vi "Camera_control_v4.vi"() -> ()   [LabVIEW 2018]
uses:
  System.Windows.Forms
  C:/Program Files/National Instruments/LabVIEW 2018/uc480DotNet.dll
  uc480DotNet.dll
panel:
  out "Time Stamp 5":timestamp format="%<%H:%M:%S\n%Y/%m/%d>T"
  out "Time Stamp 2":timestamp format="%<%H:%M:%S\n%Y/%m/%d>T"
  out "Boolean":bool
  out "?":u8(slide) scale=0.0..1.0
  in  "Capture Period (hours) 2":dbl=0.005
  in  "stop":bool
  out "Image":picture
  in  "Capture Frequency (minutes)":dbl=0.5
  out "Time Stamp":timestamp format="%<%H:%M:%S\n%Y/%m/%d>T"
  in  "Name of Operator":string="AT"
  in  "Parent Folder":path=path "D:/Dropbox (MIT)/Buonassisi-Group/AMD Team/Campaign 2.0/Degradation"
  in  "Zoom":u16(ring)=1 items=["4X"=4, "2X"=2, "1X"=1]
  in  "PictureBox":refnum<k24>(container)
  out "Serial Number 2":string
  out "Height 2":i32=8
  out "Width 2":i32=8
  out "Bits/Pixel 2":i32=8
  in  "Camera ID":i32
  out "Serial Number":string
  out "Height":i32=8
  out "Width":i32=8
  out "Bits/Pixel":i32=8
  in  "Pixelclock":i32(slide)=33 min=5 max=40 step=1 scale=5.0..40.0
  in  "Framerate":dbl(slide)=33.21525 min=0.47411700449083627 max=15.001275108384213 step=0.014032998230479876 scale=0.47411700449083627..15.001275108384213 scale format="%#.3g"
  in  "Exposure":dbl(slide)=33.21525 min=0.06241666666666667 max=99.86666666666667 step=0.06241666666666667 scale=0.06241666666666667..99.86666666666667 scale format="%#.3g"
  out "Error Out":errorcluster caption="error"
  in  "Load Parameter":bool
  in  "Exit Camera":bool
  in  "Stop Live":bool
  in  "Start Live":bool
  in  "Init Camera":bool
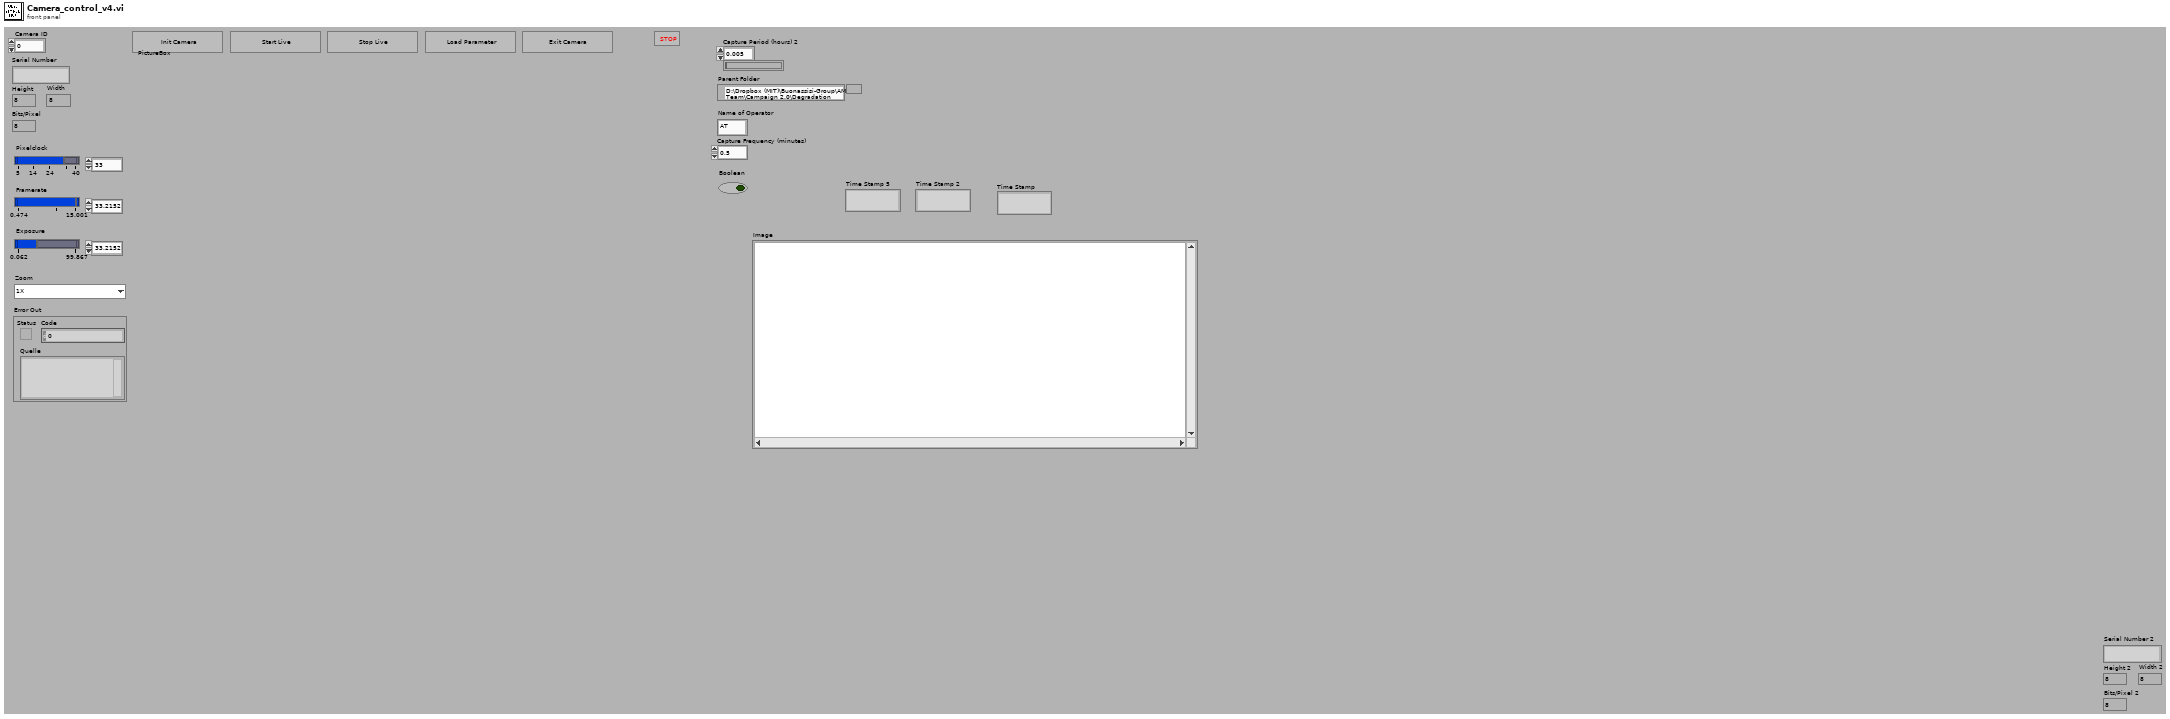
[diagram p1: front panel]
types:
  T1 = enum8{"Enabled", "Disabled", "Disabled and Grayed Out"}
  T2 = typedef "imagedata.ctl" = cluster{"image type":i32, "image depth":i32, "image":u8[], "mask":u8[], "colors":u32[], "Rectangle":cluster{"left":i16, "top":i16, "right":i16, "bottom":i16}}
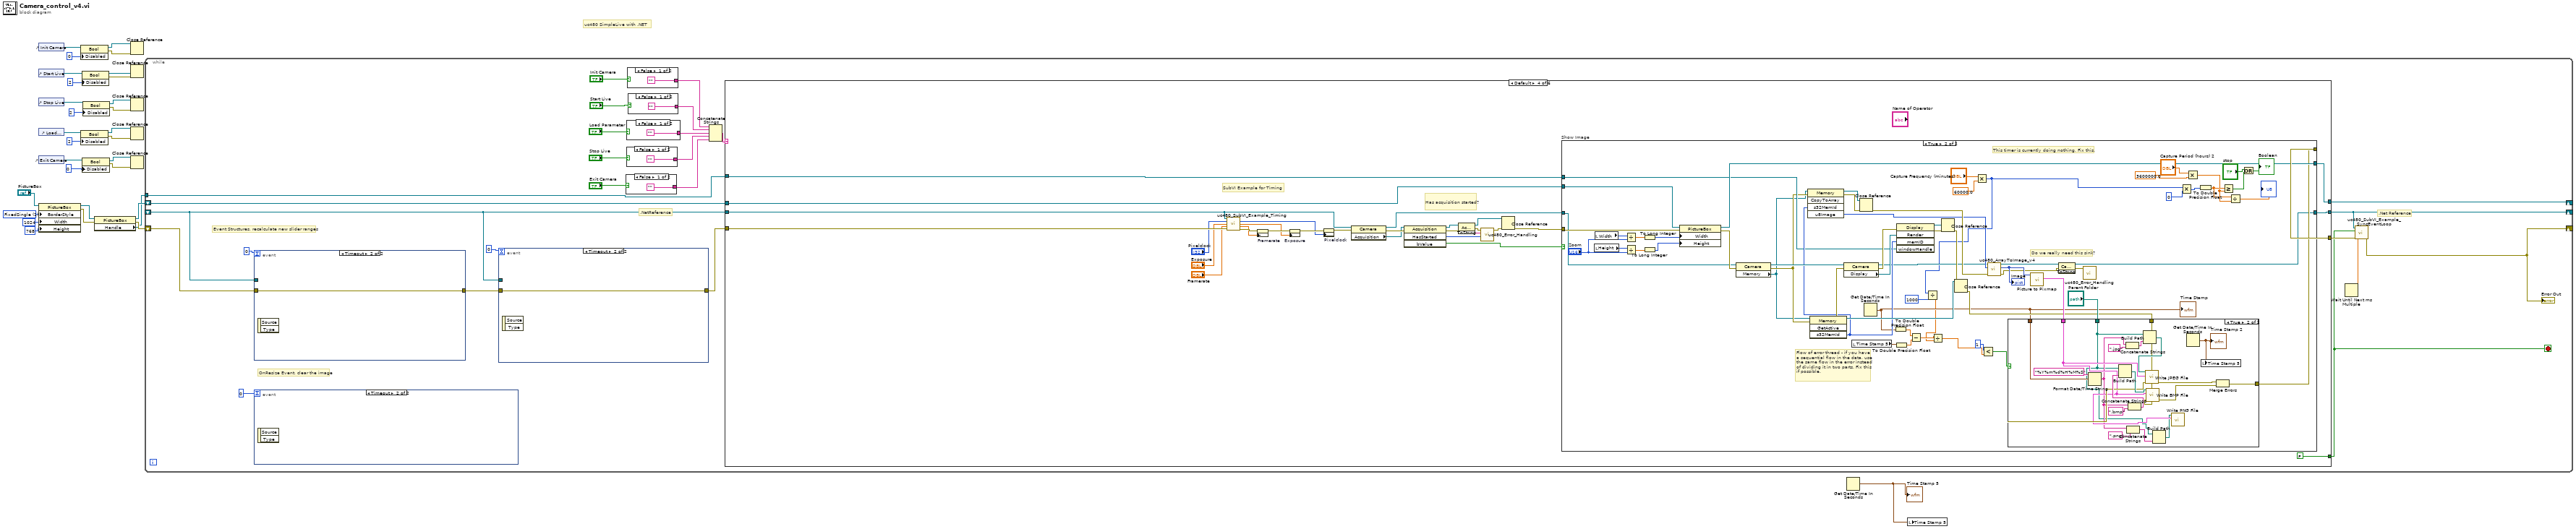
[diagram p0: block diagram]
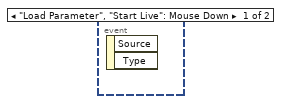
[diagram p2: hidden frame]
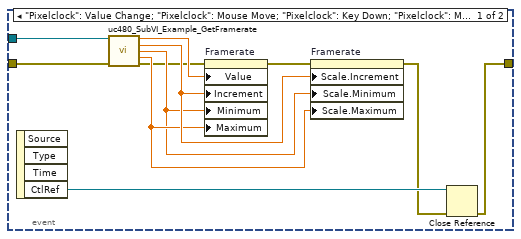
[diagram p3: hidden frame]
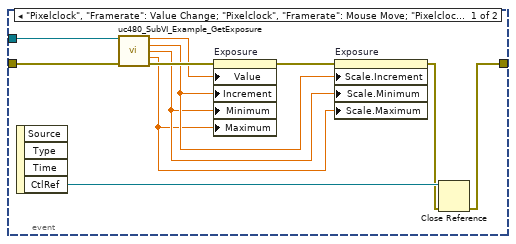
[diagram p4: hidden frame]
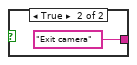
[diagram p5: hidden frame]
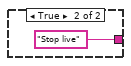
[diagram p6: hidden frame]
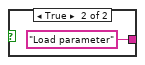
[diagram p7: hidden frame]
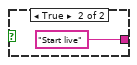
[diagram p8: hidden frame]
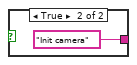
[diagram p9: hidden frame]
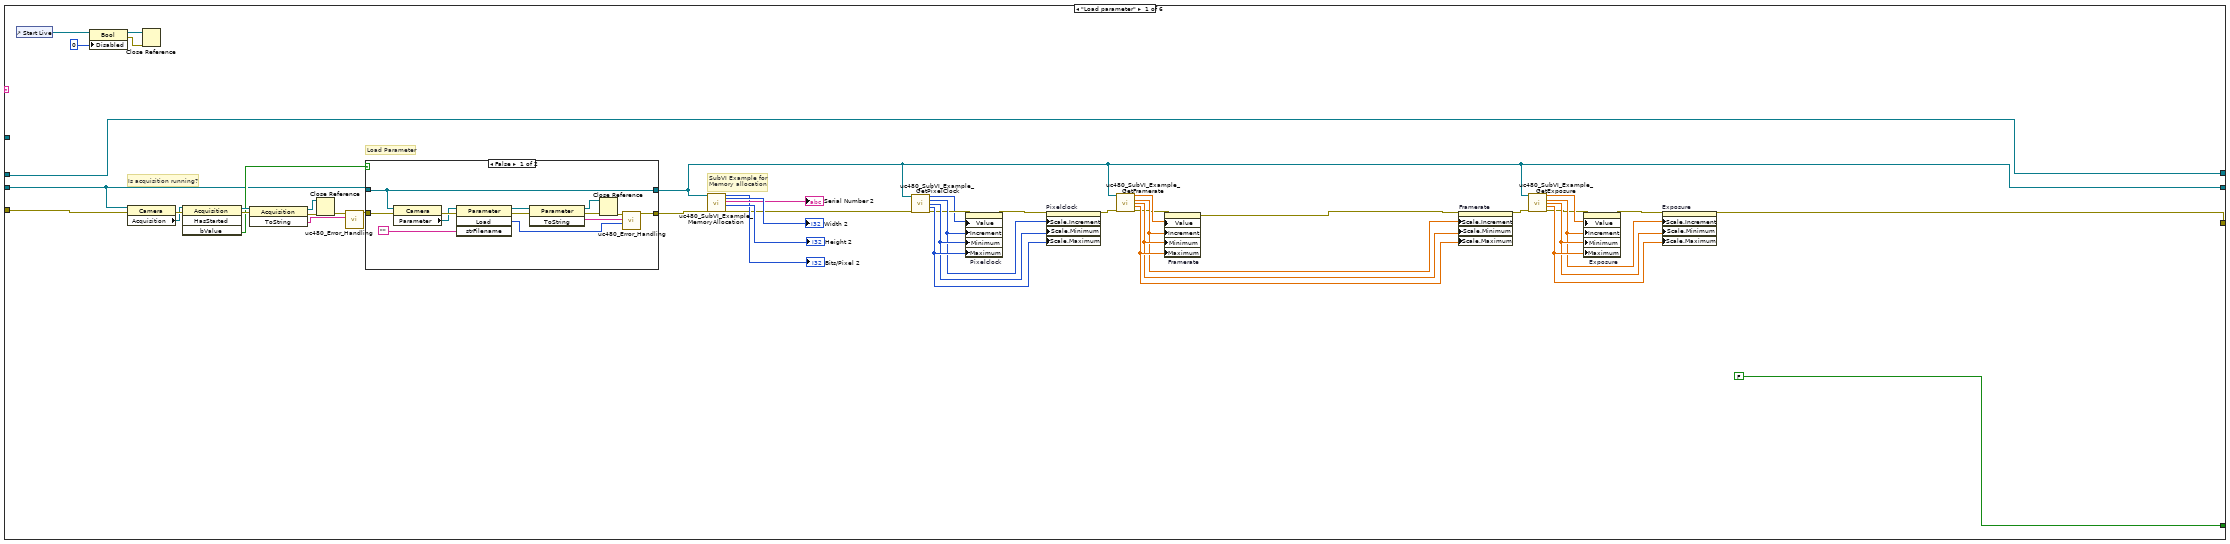
[diagram p10: hidden frame]
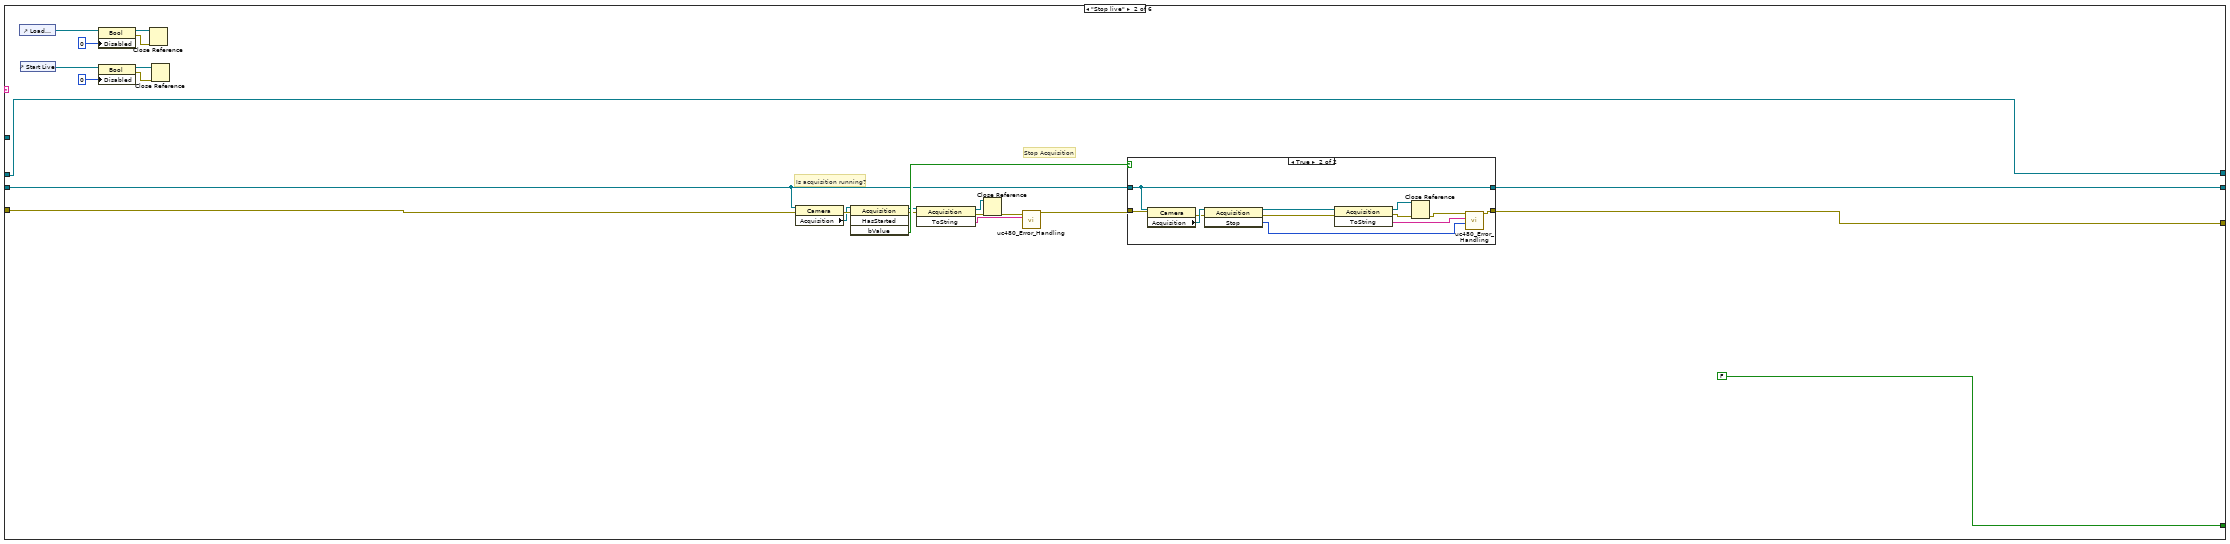
[diagram p12: hidden frame]
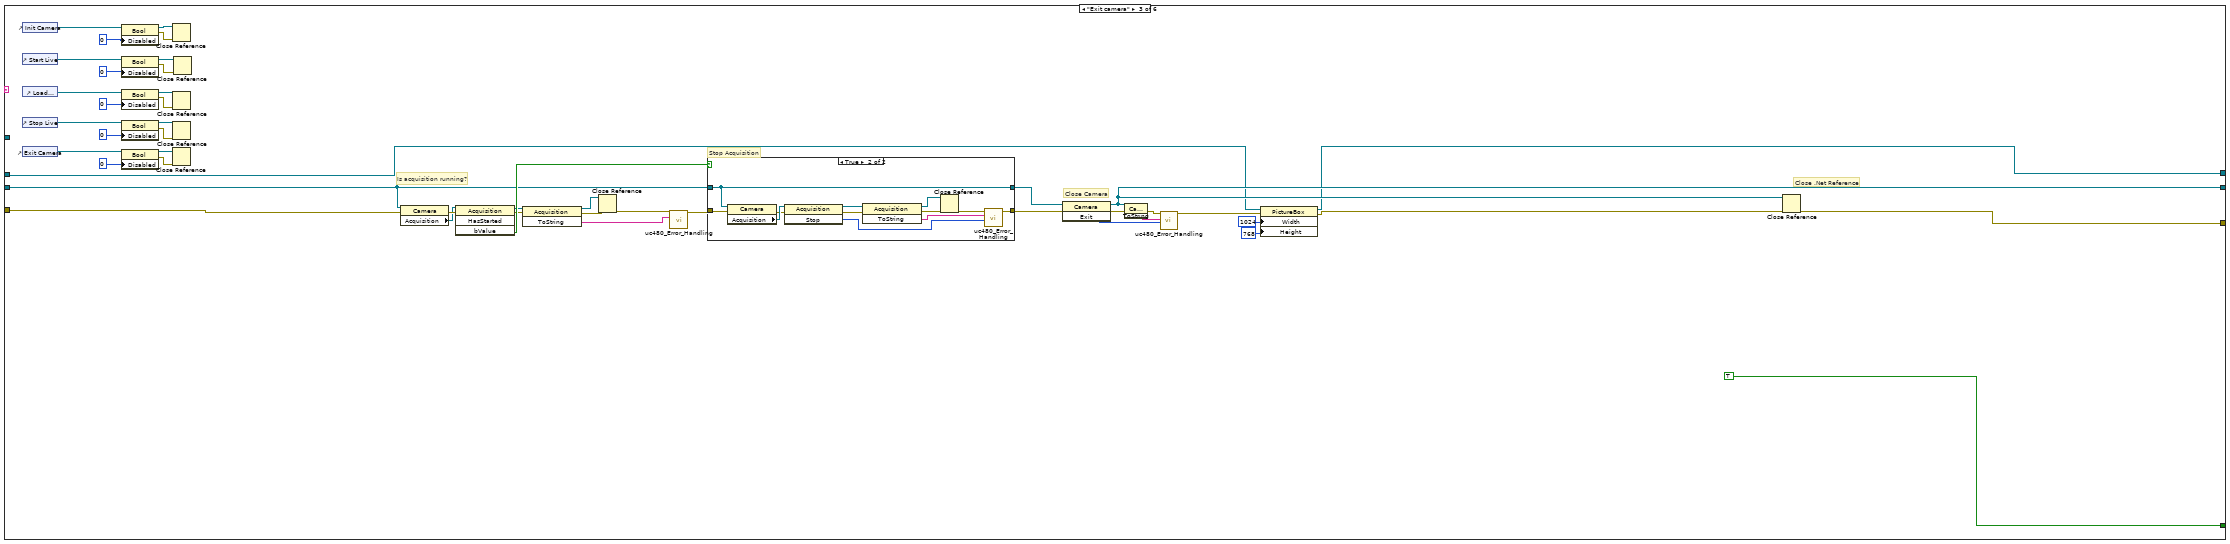
[diagram p14: hidden frame]
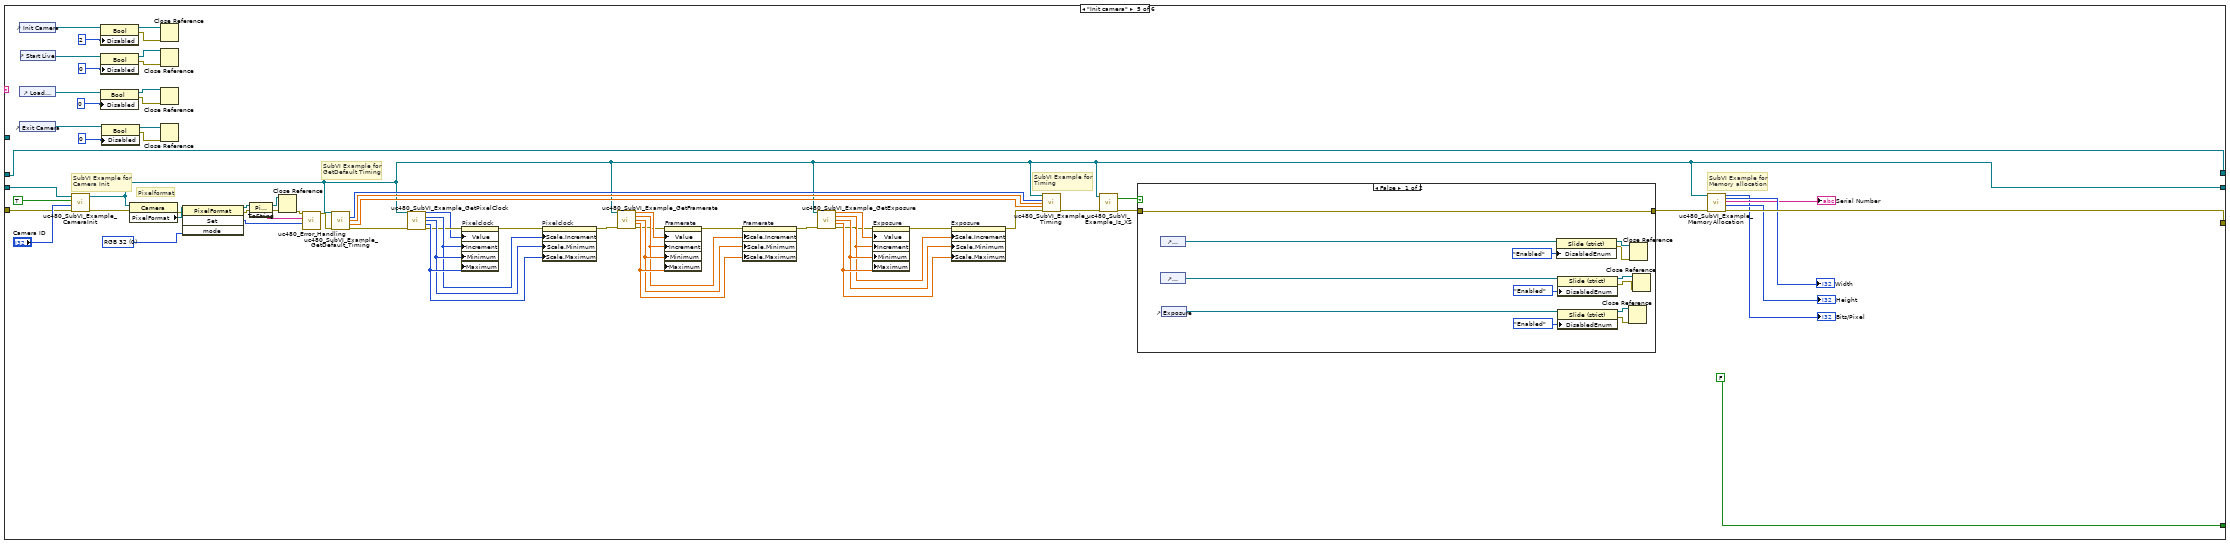
[diagram p18: hidden frame]
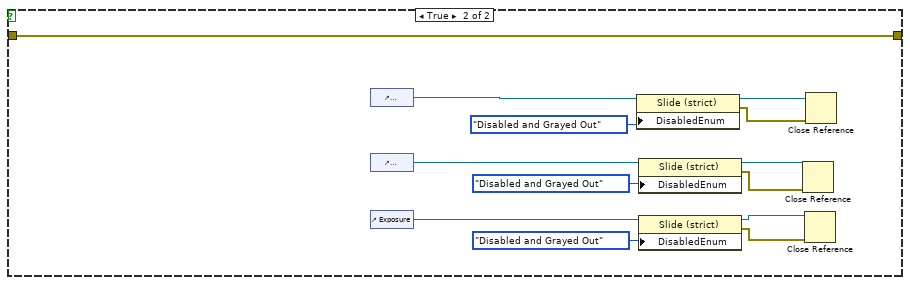
[diagram p19: hidden frame]
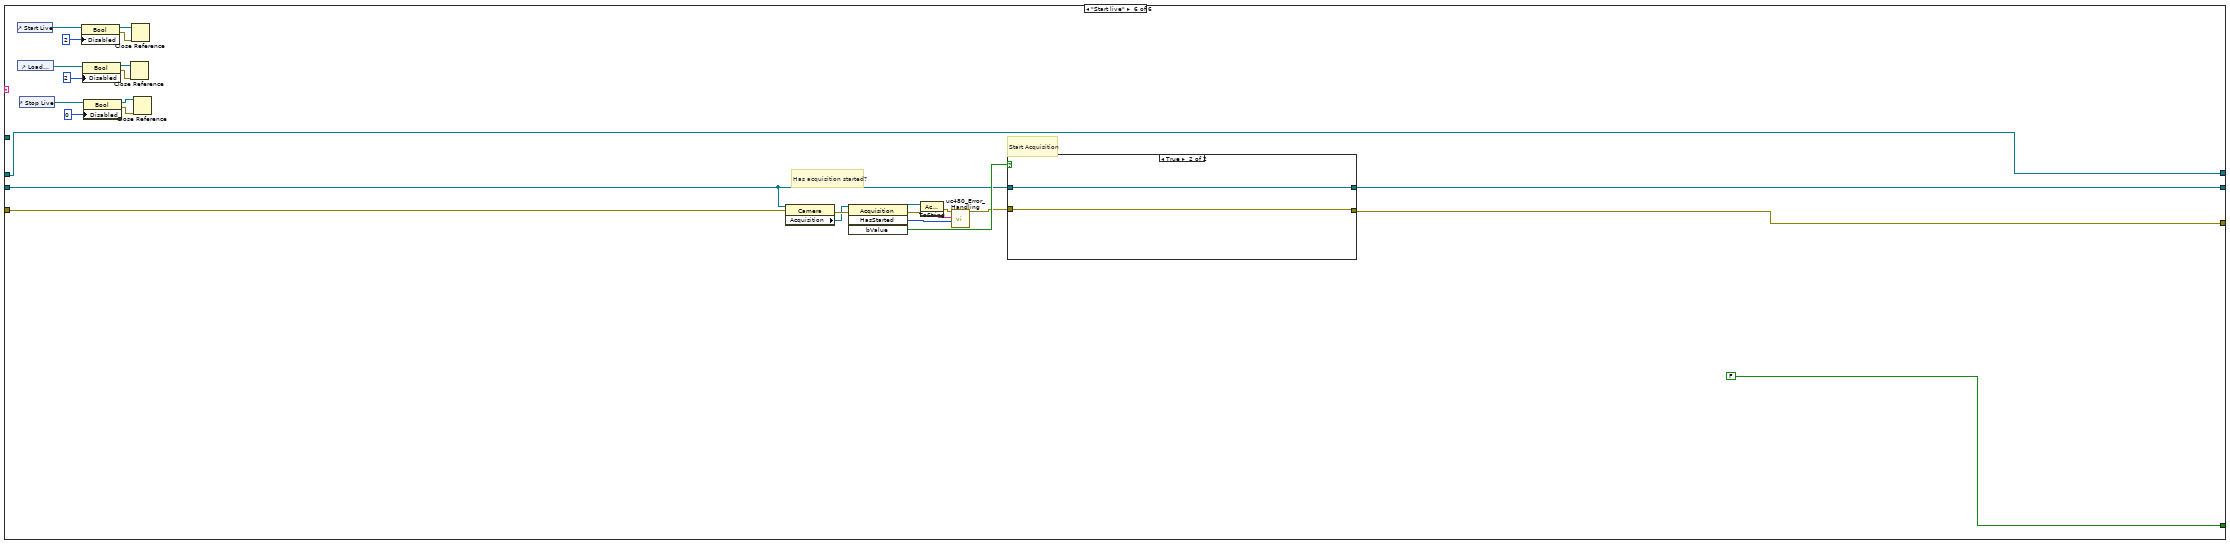
[diagram p20: hidden frame]
diagram:
  w19 = 1 items=["None", "FixedSingle", "Fixed3D"] ("BorderStyle")
  # "uc480 SimpleLive with .NET"
  n1 = control-ref of="Init Camera"() -> (w30:refnum<vi>)
  n2 = control-ref of="Start Live"() -> (w27:refnum<vi>)
  n3 = control-ref of="Stop Live"() -> (w21:refnum<vi>)
  n4 = control-ref of="Load Parameter"() -> (w22:refnum<vi>)
  n5 = control-ref of="Exit Camera"() -> (w23:refnum<vi>)
  n6 = property class="PictureBox"(reference="PictureBox", "BorderStyle"=w19, "Width"=1024, "Height"=768) -> (reference out=w5:refnum<k24>, error out=w6:errorcluster)  [unwired: 1 in]
  n7 = property class="Bool"(reference=w30, "Disabled"=u8 0 ("Deaktiviert")) -> (reference out=w16:refnum<vi>, error out=w15:errorcluster)  [unwired: 1 in]
  n8 = property class="Bool"(reference=w22, "Disabled"=u8 2 ("Deaktiviert")) -> (reference out=w10:refnum<vi>, error out=w9:errorcluster)  [unwired: 1 in]
  n9 = property class="Bool"(reference=w27, "Disabled"=u8 2 ("Deaktiviert")) -> (reference out=w14:refnum<vi>, error out=w13:errorcluster)  [unwired: 1 in]
  n10 = property class="Bool"(reference=w23, "Disabled"=u8 0 ("Deaktiviert")) -> (reference out=w8:refnum<vi>, error out=w7:errorcluster)  [unwired: 1 in]
  n11 = property class="Bool"(reference=w21, "Disabled"=u8 2 ("Deaktiviert")) -> (reference out=w12:refnum<vi>, error out=w11:errorcluster)  [unwired: 1 in]
  n12 = property class="PictureBox"(reference=w5, error in=w6) -> (reference out=w4:refnum<k24>, error out=w3:errorcluster, "Handle"=w2:refnum<k24>)
  n13 = Close Reference(reference=w16, error in (no error)=w15) -> ()  [unwired: 1 out]
  n14 = Close Reference(reference=w14, error in (no error)=w13) -> ()  [unwired: 1 out]
  n15 = Close Reference(reference=w12, error in (no error)=w11) -> ()  [unwired: 1 out]
  n16 = Close Reference(reference=w10, error in (no error)=w9) -> ()  [unwired: 1 out]
  n17 = Close Reference(reference=w8, error in (no error)=w7) -> ()  [unwired: 1 out]
  n18 = while {
    shift-right: [w36] -> _
    shift-left: w3 -> [w41]
    shift-right: [w39] -> _
    shift-left: _ -> [w32]
    shift-right: [w34] -> _
    shift-left: w4 -> [w35]
    tunnel: w2 -> [w33]
    stop <- w31 stop-if-true
    # "OnResize Event, clear the image"
    # "Event Structures, recalculate new slider ranges"
    # ".NetReference"
    # ".Net Reference"
    n19 = event shown="[1] Timeout" {
      selector: _ -> [_ _]
      dyn-events: _ -> [_ _]
      timeout: 0 -> [_ _]
      tunnel: [w57 w68] -> w42
      tunnel: w41 -> [w67 w68]
      tunnel: w32 -> [w66 _]
      event "Pixelclock": Value Change; "Pixelclock": Mouse Move; "Pixelclock": Key Down; "Pixelclock": Mouse Up {
        n20 = event-data() -> ("CtlRef"=w59:refnum<vi>)  [unwired: 1 in, 3 out]
        n21 = call <instrlib>:"uc480_SubVI_Example_GetFramerate.vi"(".NET (Reference)"=w66, "Error In"=w67) -> ("Framerate"=w65:dbl, "Inc"=w64:dbl, "Min"=w62:dbl, "Max"=w63:dbl, "error out"=w61:errorcluster)  [unwired: 9 in]
        n22 = property on="Framerate" class="Slide (strict)"(error in=w61, "Value"=w65, "Increment"=w64, "Minimum"=w62, "Maximum"=w63) -> (error out=w60:errorcluster)  [unwired: 1 in, 1 out]
        n23 = property on="Framerate" class="Slide (strict)"(error in=w60, "Scale.Increment"=w64, "Scale.Minimum"=w62, "Scale.Maximum"=w63) -> (error out=w58:errorcluster)  [unwired: 1 in, 1 out]
        n24 = Close Reference(reference=w59, error in (no error)=w58) -> (error out=w57:errorcluster)
      }
      event Timeout {
        n25 = event-data() -> ()  [unwired: 1 in, 2 out]
      }
    }
    n26 = event shown="[1] Timeout" {
      selector: _ -> [_ _]
      dyn-events: _ -> [_ _]
      timeout: 0 -> [_ _]
      event "Load Parameter", "Start Live": Mouse Down {
        n27 = event-data() -> ()  [unwired: 1 in, 2 out]
      }
      event Timeout {
        n28 = event-data() -> ()  [unwired: 1 in, 2 out]
      }
    }
    n29 = event shown="[1] Timeout" {
      selector: _ -> [_ _]
      dyn-events: _ -> [_ _]
      timeout: 0 -> [_ _]
      tunnel: w42 -> [w79 w80]
      tunnel: [w69 w80] -> w44
      tunnel: w32 -> [w78 _]
      event "Pixelclock", "Framerate": Value Change; "Pixelclock", "Framerate": Mouse Move; "Pixelclock", "Framerate": Key Down; "Pixelclock", "Framerate": Mouse Up {
        n30 = event-data() -> ("CtlRef"=w71:refnum<vi>)  [unwired: 1 in, 3 out]
        n31 = call <instrlib>:"uc480_SubVI_Example_GetExposure.vi"(".NET (Reference)"=w78, "Error In"=w79) -> ("Exposure"=w75:dbl, "Inc"=w74:dbl, "Min"=w73:dbl, "Max"=w72:dbl, "Error out"=w76:errorcluster)  [unwired: 9 in]
        n32 = property on="Exposure" class="Slide (strict)"(error in=w76, "Value"=w75, "Increment"=w74, "Minimum"=w73, "Maximum"=w72) -> (error out=w77:errorcluster)  [unwired: 1 in, 1 out]
        n33 = property on="Exposure" class="Slide (strict)"(error in=w77, "Scale.Increment"=w74, "Scale.Minimum"=w73, "Scale.Maximum"=w72) -> (error out=w70:errorcluster)  [unwired: 1 in, 1 out]
        n34 = Close Reference(reference=w71, error in (no error)=w70) -> (error out=w69:errorcluster)
      }
      event Timeout {
        n35 = event-data() -> ()  [unwired: 1 in, 2 out]
      }
    }
    n36 = case shown="False" "Exit Camera" {
      tunnel: ["" "Exit camera"] -> w46
      frame False {
      }
      frame True {
      }
    }
    n37 = case shown="False" "Load Parameter" {
      tunnel: ["" "Load parameter"] -> w50
      frame False {
      }
      frame True {
      }
    }
    n38 = case shown="False" "Stop Live" {
      tunnel: ["" "Stop live"] -> w49
      frame False {
      }
      frame True {
      }
    }
    n39 = case shown="False" "Init Camera" {
      tunnel: ["" "Init camera"] -> w54
      frame False {
      }
      frame True {
      }
    }
    n40 = case shown="False" "Start Live" {
      tunnel: ["" "Start live"] -> w53
      frame False {
      }
      frame True {
      }
    }
    n41 = Concatenate Strings(w54, w53, w50, w49, w46) -> (w52:string)
    n42 = case shown="Default" w52 {
      tunnel: w32 -> [w127 w167 w221 w263 w425 w476]
      tunnel: w44 -> [w130 w168 w222 w273 w424 w477]
      tunnel: [w97 w166 w230 w272 w381 w475] -> w39
      tunnel: [w98 w165 w231 w271 w420 w473] -> w38
      tunnel: [FALSE FALSE TRUE FALSE FALSE FALSE] -> w31
      tunnel: w35 -> [w96 w159 w201 w255 w376 w466]
      tunnel: [w96 w159 w200 w254 w376 w466] -> w34
      tunnel: w33 -> [_ _ _ w251 _ _]
      frame "Load parameter" {
        # "SubVI Example for \nMemory allocation"
        # "Is acquisition running?"
        # "Load Parameter"
        n43 = control-ref of="Start Live"() -> (w121:refnum<vi>)
        n44 = property class="Bool"(reference=w121, "Disabled"=u8 0 ("Deaktiviert")) -> (reference out=w95:refnum<vi>, error out=w94:errorcluster)  [unwired: 1 in]
        n45 = property class="Camera"(reference=w127, error in=w130) -> (error out=w135:errorcluster, "Acquisition"=w134:refnum<k24>)  [unwired: 1 out]
        n46 = Close Reference(reference=w95, error in (no error)=w94) -> ()  [unwired: 1 out]
        n47 = invoke class="Acquisition" method="HasStarted"(reference=w134, error in=w135) -> (reference out=w131:refnum<k24>, error out=w133:errorcluster, "bValue"=w129:bool)  [unwired: 2 in, 1 out]
        n48 = invoke class="Acquisition" method="ToString"(reference=w131, error in=w133) -> (reference out=w93:refnum<k24>, error out=w92:errorcluster, "ToString"=w132:string)  [unwired: 1 in]
        n49 = Close Reference(reference=w93, error in (no error)=w92) -> (error out=w91:errorcluster)
        n50 = call <instrlib>:"uc480_Error_Handling.vi"("Error String"=w132, "Error In"=w91) -> ("Error Out"=w128:errorcluster)  [unwired: 9 in]
        n51 = case shown="False" w129 {
          tunnel: w128 -> [w143 w150]
          tunnel: w127 -> [w141 w151]
          tunnel: [w142 w150] -> w122
          tunnel: [w141 w151] -> w97
          frame False {
            n52 = property class="Camera"(reference=w141, error in=w143) -> (error out=w145:errorcluster, "Parameter"=w144:refnum<k24>)  [unwired: 1 out]
            n53 = invoke class="Parameter" method="Load"(reference=w144, error in=w145, "strFilename"="") -> (reference out=w147:refnum<k24>, error out=w148:errorcluster, "Load"=w140:i32)  [unwired: 1 in, 1 out]
            n54 = invoke class="Parameter" method="ToString"(reference=w147, error in=w148) -> (reference out=w137:refnum<k24>, error out=w139:errorcluster, "ToString"=w149:string)  [unwired: 1 in]
            n55 = Close Reference(reference=w137, error in (no error)=w139) -> (error out=w138:errorcluster)
            n56 = call <instrlib>:"uc480_Error_Handling.vi"("Error Code"=w140, "Error String"=w149, "Error In"=w138) -> ("Error Out"=w142:errorcluster)  [unwired: 8 in]
          }
          frame True {
          }
        }
        n57 = call <instrlib>:"uc480_SubVI_Example_MemoryAllocation.vi"(".NET (Reference)"=w97, "Error In"=w122) -> ("Bits/Pixel 2"=→"Bits/Pixel 2":i32, "Width"=→"Width 2":i32, "Serial Number"=→"Serial Number 2":string, "Height"=→"Height 2":i32, "Error Out"=w99:errorcluster)  [unwired: 13 in]
        n58 = call <instrlib>:"uc480_SubVI_Example_GetPixelClock.vi"(".NET (Reference)"=w97, "Error In"=w99) -> ("Pixel Clock"=w100:i32, "Inc"=w102:i32, "Min"=w103:i32, "Max"=w104:i32, "error out"=w101:errorcluster)  [unwired: 9 in]
        n59 = property on="Pixelclock" class="Slide (strict)"(error in=w101, "Value"=w100, "Increment"=w102, "Minimum"=w103, "Maximum"=w104) -> (error out=w105:errorcluster)  [unwired: 1 in, 1 out]
        n60 = property on="Pixelclock" class="Slide (strict)"(error in=w105, "Scale.Increment"=w102, "Scale.Minimum"=w103, "Scale.Maximum"=w104) -> (error out=w106:errorcluster)  [unwired: 1 in, 1 out]
        n61 = call <instrlib>:"uc480_SubVI_Example_GetFramerate.vi"(".NET (Reference)"=w97, "Error In"=w106) -> ("Framerate"=w109:dbl, "Inc"=w110:dbl, "Min"=w111:dbl, "Max"=w112:dbl, "error out"=w108:errorcluster)  [unwired: 9 in]
        n62 = property on="Framerate" class="Slide (strict)"(error in=w108, "Value"=w109, "Increment"=w110, "Minimum"=w111, "Maximum"=w112) -> (error out=w107:errorcluster)  [unwired: 1 in, 1 out]
        n63 = property on="Framerate" class="Slide (strict)"(error in=w107, "Scale.Increment"=w110, "Scale.Minimum"=w111, "Scale.Maximum"=w112) -> (error out=w113:errorcluster)  [unwired: 1 in, 1 out]
        n64 = call <instrlib>:"uc480_SubVI_Example_GetExposure.vi"(".NET (Reference)"=w97, "Error In"=w113) -> ("Exposure"=w116:dbl, "Inc"=w117:dbl, "Min"=w118:dbl, "Max"=w119:dbl, "Error out"=w114:errorcluster)  [unwired: 9 in]
        n65 = property on="Exposure" class="Slide (strict)"(error in=w114, "Value"=w116, "Increment"=w117, "Minimum"=w118, "Maximum"=w119) -> (error out=w115:errorcluster)  [unwired: 1 in, 1 out]
        n66 = property on="Exposure" class="Slide (strict)"(error in=w115, "Scale.Increment"=w117, "Scale.Minimum"=w118, "Scale.Maximum"=w119) -> (error out=w98:errorcluster)  [unwired: 1 in, 1 out]
      }
      frame "Stop live" {
        # "Is acquisition running?"
        # "Stop Acquisition"
        n67 = control-ref of="Load Parameter"() -> (w163:refnum<vi>)
        n68 = control-ref of="Start Live"() -> (w160:refnum<vi>)
        n69 = property class="Bool"(reference=w163, "Disabled"=u8 0 ("Deaktiviert")) -> (reference out=w158:refnum<vi>, error out=w157:errorcluster)  [unwired: 1 in]
        n70 = property class="Bool"(reference=w160, "Disabled"=u8 0 ("Deaktiviert")) -> (reference out=w156:refnum<vi>, error out=w155:errorcluster)  [unwired: 1 in]
        n71 = Close Reference(reference=w158, error in (no error)=w157) -> ()  [unwired: 1 out]
        n72 = Close Reference(reference=w156, error in (no error)=w155) -> ()  [unwired: 1 out]
        n73 = property class="Camera"(reference=w167, error in=w168) -> (error out=w175:errorcluster, "Acquisition"=w174:refnum<k24>)  [unwired: 1 out]
        n74 = invoke class="Acquisition" method="HasStarted"(reference=w174, error in=w175) -> (reference out=w169:refnum<k24>, error out=w171:errorcluster, "bValue"=w173:bool)  [unwired: 2 in, 1 out]
        n75 = invoke class="Acquisition" method="ToString"(reference=w169, error in=w171) -> (reference out=w152:refnum<k24>, error out=w154:errorcluster, "ToString"=w170:string)  [unwired: 1 in]
        n76 = Close Reference(reference=w152, error in (no error)=w154) -> (error out=w153:errorcluster)
        n77 = call <instrlib>:"uc480_Error_Handling.vi"("Error String"=w170, "Error In"=w153) -> ("Error Out"=w172:errorcluster)  [unwired: 9 in]
        n78 = case shown="True" w173 {
          tunnel: [w177 w188] -> w165
          tunnel: w172 -> [w177 w189]
          tunnel: w167 -> [w176 w181]
          tunnel: [w176 w181] -> w166
          frame False {
          }
          frame True {
            n79 = property class="Camera"(reference=w181, error in=w189) -> (error out=w185:errorcluster, "Acquisition"=w186:refnum<k24>)  [unwired: 1 out]
            n80 = invoke class="Acquisition" method="Stop"(reference=w186, error in=w185) -> (reference out=w183:refnum<k24>, error out=w184:errorcluster, "Stop"=w182:i32)  [unwired: 1 in]
            n81 = invoke class="Acquisition" method="ToString"(reference=w183, error in=w184) -> (reference out=w178:refnum<k24>, error out=w180:errorcluster, "ToString"=w187:string)  [unwired: 1 in]
            n82 = Close Reference(reference=w178, error in (no error)=w180) -> (error out=w179:errorcluster)
            n83 = call <instrlib>:"uc480_Error_Handling.vi"("Error Code"=w182, "Error String"=w187, "Error In"=w179) -> ("Error Out"=w188:errorcluster)  [unwired: 8 in]
          }
        }
      }
      frame "Exit camera" {
        # "Close .Net Reference"
        # "Is acquisition running?"
        # "Stop Acquisition"
        # "Close Camera"
        n84 = control-ref of="Init Camera"() -> (w213:refnum<vi>)
        n85 = control-ref of="Start Live"() -> (w212:refnum<vi>)
        n86 = control-ref of="Load Parameter"() -> (w211:refnum<vi>)
        n87 = control-ref of="Stop Live"() -> (w210:refnum<vi>)
        n88 = control-ref of="Exit Camera"() -> (w209:refnum<vi>)
        n89 = property class="Bool"(reference=w213, "Disabled"=u8 0 ("Deaktiviert")) -> (reference out=w191:refnum<vi>, error out=w190:errorcluster)  [unwired: 1 in]
        n90 = property class="Bool"(reference=w212, "Disabled"=u8 0 ("Deaktiviert")) -> (reference out=w193:refnum<vi>, error out=w192:errorcluster)  [unwired: 1 in]
        n91 = property class="Bool"(reference=w211, "Disabled"=u8 0 ("Deaktiviert")) -> (reference out=w195:refnum<vi>, error out=w194:errorcluster)  [unwired: 1 in]
        n92 = property class="Bool"(reference=w210, "Disabled"=u8 0 ("Deaktiviert")) -> (reference out=w197:refnum<vi>, error out=w196:errorcluster)  [unwired: 1 in]
        n93 = property class="Bool"(reference=w209, "Disabled"=u8 0 ("Deaktiviert")) -> (reference out=w199:refnum<vi>, error out=w198:errorcluster)  [unwired: 1 in]
        n94 = Close Reference(reference=w191, error in (no error)=w190) -> ()  [unwired: 1 out]
        n95 = Close Reference(reference=w199, error in (no error)=w198) -> ()  [unwired: 1 out]
        n96 = Close Reference(reference=w195, error in (no error)=w194) -> ()  [unwired: 1 out]
        n97 = Close Reference(reference=w197, error in (no error)=w196) -> ()  [unwired: 1 out]
        n98 = Close Reference(reference=w193, error in (no error)=w192) -> ()  [unwired: 1 out]
        n99 = property class="Camera"(reference=w221, error in=w222) -> (error out=w229:errorcluster, "Acquisition"=w228:refnum<k24>)  [unwired: 1 out]
        n100 = invoke class="Acquisition" method="HasStarted"(reference=w228, error in=w229) -> (reference out=w223:refnum<k24>, error out=w225:errorcluster, "bValue"=w227:bool)  [unwired: 2 in, 1 out]
        n101 = invoke class="Acquisition" method="ToString"(reference=w223, error in=w225) -> (reference out=w206:refnum<k24>, error out=w208:errorcluster, "ToString"=w224:string)  [unwired: 1 in]
        n102 = Close Reference ("Close Referenz")(reference=w206, error in (no error)=w208) -> (error out=w207:errorcluster)
        n103 = call <instrlib>:"uc480_Error_Handling.vi"("Error String"=w224, "Error In"=w207) -> ("Error Out"=w226:errorcluster)  [unwired: 9 in]
        n104 = case shown="True" w227 {
          tunnel: [w238 w249] -> w219
          tunnel: w226 -> [w238 w250]
          tunnel: w221 -> [w237 w242]
          tunnel: [w237 w242] -> w220
          frame False {
          }
          frame True {
            n105 = property class="Camera"(reference=w242, error in=w250) -> (error out=w246:errorcluster, "Acquisition"=w247:refnum<k24>)  [unwired: 1 out]
            n106 = invoke class="Acquisition" method="Stop"(reference=w247, error in=w246) -> (reference out=w244:refnum<k24>, error out=w245:errorcluster, "Stop"=w243:i32)  [unwired: 1 in]
            n107 = invoke class="Acquisition" method="ToString"(reference=w244, error in=w245) -> (reference out=w239:refnum<k24>, error out=w241:errorcluster, "ToString"=w248:string)  [unwired: 1 in]
            n108 = Close Reference ("Close Referenz")(reference=w239, error in (no error)=w241) -> (error out=w240:errorcluster)
            n109 = call <instrlib>:"uc480_Error_Handling.vi"("Error Code"=w243, "Error String"=w248, "Error In"=w240) -> ("Error Out"=w249:errorcluster)  [unwired: 8 in]
          }
        }
        n110 = invoke class="Camera" method="Exit"(reference=w220, error in=w219) -> (reference out=w230:refnum<k24>, error out=w233:errorcluster, "Exit"=w232:i32)  [unwired: 1 in]
        n111 = invoke class="Camera" method="ToString"(reference=w230, error in=w233) -> (error out=w234:errorcluster, "ToString"=w235:string)  [unwired: 1 in, 1 out]
        n112 = call <instrlib>:"uc480_Error_Handling.vi"("Error Code"=w232, "Error String"=w235, "Error In"=w234) -> ("Error Out"=w205:errorcluster)  [unwired: 8 in]
        n113 = property class="PictureBox"(reference=w201, error in=w205, "Width"=1024, "Height"=768) -> (reference out=w200:refnum<k24>, error out=w204:errorcluster)
        n114 = Close Reference ("Close Referenz")(reference=w230, error in (no error)=w204) -> (error out=w231:errorcluster)
      }
      frame Default {
        # "SubVI Example for Timing"
        # "Has acquisition started?"
        n115 = call <instrlib>:"uc480_SubVI_Example_Timing.vi"(".NET (Reference)"=w263, "Pixelclock"="Pixelclock", "Exposure time"="Exposure", "Framerate"="Framerate", "Error In"=w273) -> ("Pixelclock"=w266:i32, "Exposure time"=w265:dbl, "Framerate"=w264:dbl, "Error Out"=w270:errorcluster)  [unwired: 7 in]
        n116 = property on="Framerate" class="Schieber (strikt)"(error in=w270, "Scale.RngStart"=w264) -> (error out=w269:errorcluster)  [unwired: 1 in, 1 out]
        n117 = property on="Exposure" class="Schieber (strikt)"(error in=w269, "Scale.RngStart"=w265) -> (error out=w268:errorcluster)  [unwired: 1 in, 1 out]
        n118 = property on="Pixelclock" class="Schieber (strikt)"(error in=w268, "Scale.RngStart"=w266) -> (error out=w267:errorcluster)  [unwired: 1 in, 1 out]
        n119 = property class="Camera"(reference=w263, error in=w267) -> (reference out=w256:refnum<k24>, error out=w279:errorcluster, "Acquisition"=w278:refnum<k24>)
        n120 = invoke class="Acquisition" method="HasStarted"(reference=w278, error in=w279) -> (reference out=w253:refnum<k24>, error out=w275:errorcluster, "HasStarted"=w274:i32, "bValue"=w252:bool)  [unwired: 2 in]
        n121 = invoke class="Acquisition" method="ToString"(reference=w253, error in=w275) -> (reference out=w257:refnum<k24>, error out=w277:errorcluster, "ToString"=w276:string)  [unwired: 1 in]
        n122 = call <instrlib>:"uc480_Error_Handling.vi"("Error Code"=w274, "Error String"=w276, "Error In"=w277) -> ("Error Out"=w259:errorcluster)  [unwired: 8 in]
        n123 = Close Reference(reference=w257, error in (no error)=w259) -> (error out=w258:errorcluster)
        n124 = case "Show Image" shown="True" w252 {
          tunnel: [w283 w319] -> w271
          tunnel: w258 -> [w283 w340]
          tunnel: w256 -> [w282 w316]
          tunnel: [w282 w296] -> w272
          tunnel: w255 -> [w281 w341]
          tunnel: [w281 w330] -> w254
          tunnel: w251 -> [_ w324]
          frame False {
          }
          frame True {
            # "This timer is currently doing nothing. Fix this."
            # "Do we really need this sink?"
            # "Flow of error thread - if you have\na sequential flow in the data, use\nthe same flow in the error instead\nof dividing it in two parts. Fix this\nif possible."
            n125 = local read "Height"() -> (w338:i32)
            n126 = local read "Width"() -> (w334:i32)
            n127 = Divide(x=w334, y="Zoom") -> (x/y=w336:dbl)
            n128 = Divide(x=w338, y="Zoom") -> (x/y=w339:dbl)
            n129 = To Long Integer(number=w336) -> (32bit integer=w335:i32)
            n130 = To Long Integer(number=w339) -> (32bit integer=w337:i32)
            n131 = property class="PictureBox"(reference=w341, error in=w340, "Width"=w335, "Height"=w337) -> (reference out=w330:refnum<k24>, error out=w325:errorcluster)
            n132 = property class="Camera"(reference=w316, error in=w325) -> (reference out=w328:refnum<k24>, error out=w318:errorcluster, "Memory"=w317:refnum<k24>)
            n133 = invoke class="Memory" method="GetActive"(reference=w317, error in=w318) -> (reference out=w327:refnum<k24>, error out=w331:errorcluster, "s32MemId"=w326:i32)  [unwired: 2 in, 1 out]
            n134 = invoke class="Memory" method="CopyToArray"(reference=w317, error in=w318, "s32MemId"=w326) -> (reference out=w322:refnum<k24>, error out=w321:errorcluster, "u8Image"=w314:u8[])  [unwired: 2 in, 2 out]
            n135 = property class="Camera"(reference=w328, error in=w331) -> (reference out=w298:refnum<k24>, error out=w342:errorcluster, "Display"=w344:refnum<k24>)
            n136 = local read "Time Stamp 5"() -> (w284:timestamp)
            n137 = Close Reference(reference=w322, error in (no error)=w321) -> (error out=w315:errorcluster)
            n138 = Get Date/Time In Seconds() -> (seconds since 1Jan1904=w294:timestamp)
            "Time Stamp" <- w294
            n139 = To Double Precision Float(number=w294) -> (double precision float=w293:dbl)
            n140 = To Double Precision Float(number=w284) -> (double precision float=w292:dbl)
            n141 = invoke class="Display" method="Render"(reference=w344, error in=w342, "memID"=w326, "windowHandle"=w324) -> (reference out=w343:refnum<k24>, error out=w323:errorcluster)  [unwired: 1 in, 3 out]
            n142 = Subtract(x=w293, y=w292) -> (x-y=w291:dbl)
            n143 = Close Reference(reference=w343, error in (no error)=w323) -> (error out=w332:errorcluster)
            n144 = Close Reference(reference=w327, error in (no error)=w332) -> (error out=w299:errorcluster)
            n145 = Multiply(x="Capture Frequency (minutes)", y=60000.0) -> (x*y=w287:i32)
            n146 = Divide(x=w287, y=1000) -> (x/y=w285:dbl)
            n147 = Divide(x=w291, y=w285) -> (x/y=w289:dbl)
            n148 = Less?(x=1, y=w289) -> (x < y?=w295:bool)
            n149 = call "uc480_ArrayToImage_v4.vi"("Error In"=w315, "InArray"=w314, ".NET (Reference)"=w298) -> ("Error Out"=w302:errorcluster, "Image"=w304:picture, ".NET (Reference) 2"=w297:refnum<k24>)  [unwired: 6 in]
            "Image" <- w304
            n150 = call <vilib>:"Picture to Pixmap.vi"("picture"=w304) -> ("image data"=w305:T2)  [unwired: 9 in, 1 out]
            n151 = case shown="True" w295 {
              tunnel: "Parent Folder" -> [_ w347]
              tunnel: [w345 w364] -> w319
              tunnel: w294 -> [_ w360]
              tunnel: w305 -> [_ w351]
              tunnel: w299 -> [w345 w353]
              frame False {
              }
              frame True {
                n152 = Format Date/Time String(time format string (%c)="%Y%m%d%H%M%S", seconds (now)=w360) -> (date/time string=w349:string)  [unwired: 1 in]
                n153 = Concatenate Strings(w349, ".jpg") -> (w358:string)
                n154 = Concatenate Strings(w349, ".png") -> (w348:string)
                n155 = Concatenate Strings(w349, ".bmp") -> (w354:string)
                n156 = Build Path(base path=w347, name or relative path=w354) -> (appended path=w356:path)
                n157 = Build Path(base path=w347, name or relative path=w358) -> (appended path=w357:path)
                n158 = call <vilib>:"Write JPEG File.vi"("error in (no error)"=w353, "image data"=w351, "path to JPEG file"=w357) -> ("error out"=w361:errorcluster)  [unwired: 7 in, 1 out]
                n159 = call <vilib>:"Write BMP File.vi"("error in (no error)"=w353, "image data"=w351, "path to BMP file"=w356) -> ("error out"=w362:errorcluster)  [unwired: 7 in, 1 out]
                n160 = Build Path(base path=w347, name or relative path=w348) -> (appended path=w346:path)
                n161 = call <vilib>:"Write PNG File.vi"("image data"=w351, "path to PNG file"=w346) -> ()  [unwired: 8 in, 2 out]
                n162 = Get Date/Time In Seconds() -> (seconds since 1Jan1904=w352:timestamp)
                "Time Stamp 2" <- w352
                n163 = local write "Time Stamp 5"(w352) -> ()
                n164 = Merge Errors(w361, w362) -> (w364:errorcluster)
              }
            }
            n165 = invoke class="Camera" method="ToString"(reference=w297, error in=w302) -> (reference out=w296:refnum<k24>, error out=w303:errorcluster)  [unwired: 1 in, 1 out]
            n166 = call <instrlib>:"uc480_Error_Handling.vi"("Error In"=w303) -> ()  [unwired: 10 in, 1 out]
            n167 = Multiply(x=w287, y=0) -> (x*y=w313:i32)
            n168 = Multiply(x="Capture Period (hours) 2", y=3600000.0) -> (x*y=w309:dbl)
            n169 = To Double Precision Float(number=w313) -> (double precision float=w310:dbl)
            n170 = Greater Or Equal?(x=w310, y=w309) -> (x >= y?=w307:bool)
            n171 = Divide(x=w310, y=w309) -> (x/y=→"?":dbl)
            n172 = Or(x="stop", y=w307) -> (x .or. y?=→"Boolean":bool)
          }
        }
      }
      frame "Init camera" {
        w433 = 0 items=["RGB 32"=0, "RGB 24"=1, "Y8 Monochrom"=6] ("Mode")
        # "SubVI Example for \nGetDefault Timing"
        # "SubVI Example for \nMemory allocation"
        # "SubVI Example for \nTiming"
        # "SubVI Example for \nCamera Init"
        # "Pixelformat"
        n173 = control-ref of="Init Camera"() -> (w388:refnum<vi>)
        n174 = control-ref of="Load Parameter"() -> (w384:refnum<vi>)
        n175 = control-ref of="Exit Camera"() -> (w382:refnum<vi>)
        n176 = control-ref of="Start Live"() -> (w386:refnum<vi>)
        n177 = call <instrlib>:"uc480_SubVI_Example_CameraInit.vi"("Error In"=w424, "Camera ID"="Camera ID", "Init Camera Flag"=TRUE, ".NET (Reference)"=w425) -> ("Error Out"=w430:errorcluster, ".NET (Reference)"=w381:refnum<k24>)  [unwired: 6 in]
        n178 = property class="Bool"(reference=w384, "Disabled"=u8 0 ("Deaktiviert")) -> (reference out=w371:refnum<vi>, error out=w370:errorcluster)  [unwired: 1 in]
        n179 = property class="Bool"(reference=w388, "Disabled"=u8 2 ("Deaktiviert")) -> (reference out=w375:refnum<vi>, error out=w374:errorcluster)  [unwired: 1 in]
        n180 = property class="Bool"(reference=w386, "Disabled"=u8 0 ("Deaktiviert")) -> (reference out=w373:refnum<vi>, error out=w372:errorcluster)  [unwired: 1 in]
        n181 = property class="Bool"(reference=w382, "Disabled"=u8 0 ("Deaktiviert")) -> (reference out=w369:refnum<vi>, error out=w368:errorcluster)  [unwired: 1 in]
        n182 = property on="Property Node" class="Camera"(reference=w381, error in=w430) -> (error out=w431:errorcluster, "PixelFormat"=w432:refnum<k24>)  [unwired: 1 out]
        n183 = Close Reference(reference=w375, error in (no error)=w374) -> ()  [unwired: 1 out]
        n184 = Close Reference(reference=w373, error in (no error)=w372) -> ()  [unwired: 1 out]
        n185 = Close Reference(reference=w371, error in (no error)=w370) -> ()  [unwired: 1 out]
        n186 = Close Reference(reference=w369, error in (no error)=w368) -> ()  [unwired: 1 out]
        n187 = invoke class="PixelFormat" method="Set"(reference=w432, error in=w431, "mode"=w433) -> (reference out=w428:refnum<k24>, error out=w421:errorcluster, "Set"=w427:i32)  [unwired: 1 in, 1 out]
        n188 = invoke class="PixelFormat" method="ToString"(reference=w428, error in=w421) -> (reference out=w365:refnum<k24>, error out=w367:errorcluster, "ToString"=w429:string)  [unwired: 1 in]
        n189 = Close Reference(reference=w365, error in (no error)=w367) -> (error out=w366:errorcluster)
        n190 = call <instrlib>:"uc480_Error_Handling.vi"("Error Code"=w427, "Error String"=w429, "Error In"=w366) -> ("Error Out"=w395:errorcluster)  [unwired: 8 in]
        n191 = call <instrlib>:"uc480_SubVI_Example_GetDefault_Timing.vi"(".NET (Reference)"=w381, "Error In"=w395) -> ("Pixelclock"=w394:i32, "Exposure time"=w393:dbl, "Framerate"=w392:dbl, "Error Out"=w391:errorcluster)  [unwired: 10 in]
        n192 = call <instrlib>:"uc480_SubVI_Example_GetPixelClock.vi"(".NET (Reference)"=w381, "Error In"=w391) -> ("Pixel Clock"=w396:i32, "Inc"=w398:i32, "Min"=w399:i32, "Max"=w400:i32, "error out"=w397:errorcluster)  [unwired: 9 in]
        n193 = property on="Pixelclock" class="Slide (strict)"(error in=w397, "Value"=w396, "Increment"=w398, "Minimum"=w399, "Maximum"=w400) -> (error out=w401:errorcluster)  [unwired: 1 in, 1 out]
        n194 = property on="Pixelclock" class="Slide (strict)"(error in=w401, "Scale.Increment"=w398, "Scale.Minimum"=w399, "Scale.Maximum"=w400) -> (error out=w402:errorcluster)  [unwired: 1 in, 1 out]
        n195 = call <instrlib>:"uc480_SubVI_Example_GetFramerate.vi"(".NET (Reference)"=w381, "Error In"=w402) -> ("Framerate"=w405:dbl, "Inc"=w406:dbl, "Min"=w407:dbl, "Max"=w408:dbl, "error out"=w404:errorcluster)  [unwired: 9 in]
        n196 = property on="Framerate" class="Slide (strict)"(error in=w404, "Value"=w405, "Increment"=w406, "Minimum"=w407, "Maximum"=w408) -> (error out=w403:errorcluster)  [unwired: 1 in, 1 out]
        n197 = property on="Framerate" class="Slide (strict)"(error in=w403, "Scale.Increment"=w406, "Scale.Minimum"=w407, "Scale.Maximum"=w408) -> (error out=w409:errorcluster)  [unwired: 1 in, 1 out]
        n198 = call <instrlib>:"uc480_SubVI_Example_GetExposure.vi"(".NET (Reference)"=w381, "Error In"=w409) -> ("Exposure"=w412:dbl, "Inc"=w413:dbl, "Min"=w414:dbl, "Max"=w415:dbl, "Error out"=w410:errorcluster)  [unwired: 9 in]
        n199 = property on="Exposure" class="Slide (strict)"(error in=w410, "Value"=w412, "Increment"=w413, "Minimum"=w414, "Maximum"=w415) -> (error out=w411:errorcluster)  [unwired: 1 in, 1 out]
        n200 = property on="Exposure" class="Slide (strict)"(error in=w411, "Scale.Increment"=w413, "Scale.Minimum"=w414, "Scale.Maximum"=w415) -> (error out=w390:errorcluster)  [unwired: 1 in, 1 out]
        n201 = call <instrlib>:"uc480_SubVI_Example_Timing.vi"(".NET (Reference)"=w381, "Pixelclock"=w394, "Exposure time"=w393, "Framerate"=w392, "Error In"=w390) -> ("Error Out"=w380:errorcluster)  [unwired: 7 in, 3 out]
        n202 = call <instrlib>:"uc480_SubVI_Example_Is_XS.vi"("Error In"=w380, ".NET (Reference)"=w381) -> ("Error Out"=w377:errorcluster, "IsXS"=w379:bool)  [unwired: 7 in, 1 out]
        n203 = case shown="False" w379 {
          tunnel: w377 -> [w446 w459]
          tunnel: [w446 w459] -> w378
          frame False {
            n204 = control-ref of="Pixelclock"() -> (w442:refnum<vi>)
            n205 = control-ref of="Framerate"() -> (w441:refnum<vi>)
            n206 = control-ref of="Exposure"() -> (w440:refnum<vi>)
            n207 = property class="Slide (strict)"(reference=w442, "DisabledEnum"=T1."Enabled" ("Disabled")) -> (reference out=w439:refnum<vi>, error out=w438:errorcluster)  [unwired: 1 in]
            n208 = property class="Slide (strict)"(reference=w441, "DisabledEnum"=T1."Enabled" ("Disabled")) -> (reference out=w437:refnum<vi>, error out=w436:errorcluster)  [unwired: 1 in]
            n209 = property class="Slide (strict)"(reference=w440, "DisabledEnum"=T1."Enabled" ("Disabled")) -> (reference out=w435:refnum<vi>, error out=w434:errorcluster)  [unwired: 1 in]
            n210 = Close Reference(reference=w435, error in (no error)=w434) -> ()  [unwired: 1 out]
            n211 = Close Reference(reference=w439, error in (no error)=w438) -> ()  [unwired: 1 out]
            n212 = Close Reference(reference=w437, error in (no error)=w436) -> ()  [unwired: 1 out]
          }
          frame True {
            n213 = control-ref of="Pixelclock"() -> (w458:refnum<vi>)
            n214 = control-ref of="Framerate"() -> (w455:refnum<vi>)
            n215 = control-ref of="Exposure"() -> (w453:refnum<vi>)
            n216 = property class="Slide (strict)"(reference=w458, "DisabledEnum"=T1."Disabled and Grayed Out" ("Disabled")) -> (reference out=w451:refnum<vi>, error out=w452:errorcluster)  [unwired: 1 in]
            n217 = property class="Slide (strict)"(reference=w455, "DisabledEnum"=T1."Disabled and Grayed Out" ("Disabled")) -> (reference out=w450:refnum<vi>, error out=w449:errorcluster)  [unwired: 1 in]
            n218 = property class="Slide (strict)"(reference=w453, "DisabledEnum"=T1."Disabled and Grayed Out" ("Disabled")) -> (reference out=w448:refnum<vi>, error out=w447:errorcluster)  [unwired: 1 in]
            n219 = Close Reference(reference=w450, error in (no error)=w449) -> ()  [unwired: 1 out]
            n220 = Close Reference(reference=w448, error in (no error)=w447) -> ()  [unwired: 1 out]
            n221 = Close Reference(reference=w451, error in (no error)=w452) -> ()  [unwired: 1 out]
          }
        }
        n222 = call <instrlib>:"uc480_SubVI_Example_MemoryAllocation.vi"(".NET (Reference)"=w381, "Error In"=w378) -> ("Bits/Pixel 2"=→"Bits/Pixel":i32, "Width"=→"Width":i32, "Serial Number"=→"Serial Number":string, "Height"=→"Height":i32, "Error Out"=w420:errorcluster)  [unwired: 13 in]
      }
      frame "Start live" {
        # "Has acquisition started?"
        # "Start Acquisition"
        n223 = control-ref of="Start Live"() -> (w472:refnum<vi>)
        n224 = control-ref of="Load Parameter"() -> (w469:refnum<vi>)
        n225 = control-ref of="Stop Live"() -> (w467:refnum<vi>)
        n226 = property class="Bool"(reference=w472, "Disabled"=u8 2 ("Deaktiviert")) -> (reference out=w461:refnum<vi>, error out=w460:errorcluster)  [unwired: 1 in]
        n227 = property class="Bool"(reference=w469, "Disabled"=u8 2 ("Deaktiviert")) -> (reference out=w463:refnum<vi>, error out=w462:errorcluster)  [unwired: 1 in]
        n228 = property class="Bool"(reference=w467, "Disabled"=u8 0 ("Deaktiviert")) -> (reference out=w465:refnum<vi>, error out=w464:errorcluster)  [unwired: 1 in]
        n229 = Close Reference(reference=w463, error in (no error)=w462) -> ()  [unwired: 1 out]
        n230 = Close Reference(reference=w461, error in (no error)=w460) -> ()  [unwired: 1 out]
        n231 = Close Reference(reference=w465, error in (no error)=w464) -> ()  [unwired: 1 out]
        n232 = property class="Camera"(reference=w476, error in=w477) -> (error out=w486:errorcluster, "Acquisition"=w485:refnum<k24>)  [unwired: 1 out]
        n233 = invoke class="Acquisition" method="HasStarted"(reference=w485, error in=w486) -> (reference out=w481:refnum<k24>, error out=w480:errorcluster, "HasStarted"=w479:i32, "bValue"=w484:bool)  [unwired: 2 in]
        n234 = invoke class="Acquisition" method="ToString"(reference=w481, error in=w480) -> (error out=w483:errorcluster, "ToString"=w482:string)  [unwired: 1 in, 1 out]
        n235 = call <instrlib>:"uc480_Error_Handling.vi"("Error Code"=w479, "Error String"=w482, "Error In"=w483) -> ("Error Out"=w478:errorcluster)  [unwired: 8 in]
        n236 = case shown="True" w484 {
          tunnel: [w489 w499] -> w473
          tunnel: w478 -> [w495 w499]
          tunnel: w476 -> [w494 w498]
          tunnel: [w494 w498] -> w475
          frame False {
            w487 = 1 items=["IS_DONT_WAIT", "IS_WAIT"] ("Wait")
            n237 = property class="Camera"(reference=w494, error in=w495) -> (error out=w496:errorcluster, "Acquisition"=w497:refnum<k24>)  [unwired: 1 out]
            n238 = invoke class="Acquisition" method="Capture"(reference=w497, error in=w496, "param"=w487) -> (reference out=w490:refnum<k24>, error out=w491:errorcluster, "Capture"=w488:i32)  [unwired: 1 in, 1 out]
            n239 = invoke class="Acquisition" method="ToString"(reference=w490, error in=w491) -> (error out=w493:errorcluster, "ToString"=w492:string)  [unwired: 1 in, 1 out]
            n240 = call <instrlib>:"uc480_Error_Handling.vi"("Error Code"=w488, "Error String"=w492, "Error In"=w493) -> ("Error Out"=w489:errorcluster)  [unwired: 8 in]
          }
          frame True {
          }
        }
      }
    }
    n241 = call <instrlib>:"uc480_SubVI_Example_SyncEventLoop.vi"("Error In"=w38, "use sync"=w31, ".NET (Reference)"=w39) -> ("Error Out"=w36:errorcluster, "Synchronize (ms)"=w37:dbl)  [unwired: 7 in]
    "Error Out" <- w36
    n242 = Wait Until Next ms Multiple(millisecond multiple=w37) -> ()  [unwired: 1 out]
  }
  n243 = Get Date/Time In Seconds() -> (seconds since 1Jan1904=w1:timestamp)
  "Time Stamp 5" <- w1
  n244 = local write "Time Stamp 5"(w1) -> ()
